vi "FM_Unit_Conversion.vi"(10 "Input Array [A]":dbl[](array[numeric])) -> (2 "Output Array [kg/h]":dbl[](array[numeric]))   [LabVIEW 2017]
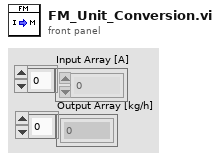
[diagram p1: front panel]
types:
  T1 = cluster{"Input Array [A][0]":dbl, "Input Array [A][1]":dbl, "Input Array [A][2]":dbl, "Input Array [A][3]":dbl}
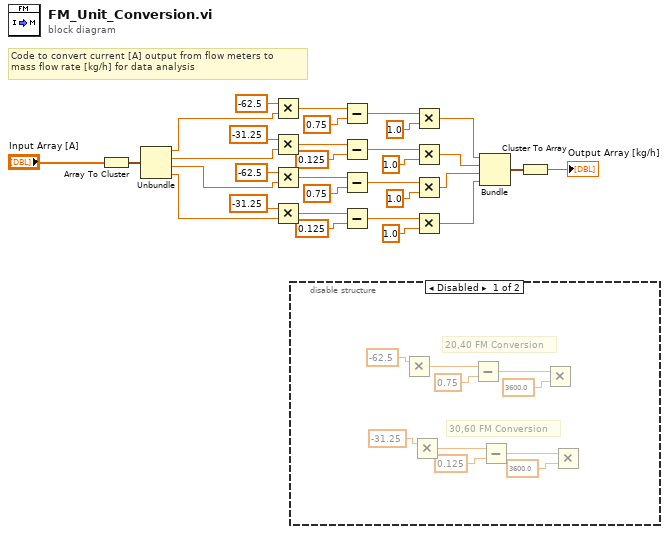
[diagram p0: block diagram]
diagram:
  # "Code to convert current [A] output from flow meters to \nmass flow rate [kg/h] for data analysis"
  n1 = Array To Cluster(array="Input Array [A]") -> (cluster=w32:T1)
  n2 = Unbundle(w32) -> ("Input Array [A][0]"=w9:dbl, "Input Array [A][1]"=w8:dbl, "Input Array [A][2]"=w7:dbl, "Input Array [A][3]"=w6:dbl)
  n3 = Multiply(x=-62.5, y=w9) -> (x*y=w28:dbl)
  n4 = Multiply(x=-31.25, y=w8) -> (x*y=w23:dbl)
  n5 = Multiply(x=-62.5, y=w7) -> (x*y=w18:dbl)
  n6 = Multiply(x=-31.25, y=w6) -> (x*y=w13:dbl)
  n7 = disable-structure shown="Disabled" {
    frame Disabled {
      # "30,60 FM Conversion"
      # "20,40 FM Conversion"
      n8 = Multiply(x=-62.5) -> (x*y=w39:dbl)  [unwired: 1 in]
      n9 = Multiply(x=-31.25) -> (x*y=w41:dbl)  [unwired: 1 in]
      n10 = Subtract(x=w39, y=0.75) -> (x-y=w40:dbl)
      n11 = Subtract(x=w41, y=0.125) -> (x-y=w42:dbl)
      n12 = Multiply(x=w40, y=3600.0) -> ()  [unwired: 1 out]
      n13 = Multiply(x=w42, y=3600.0) -> ()  [unwired: 1 out]
    }
    frame Enabled {
    }
  }
  n14 = Subtract(x=w28, y=0.75) -> (x-y=w26:dbl)
  n15 = Subtract(x=w23, y=0.125) -> (x-y=w21:dbl)
  n16 = Subtract(x=w18, y=0.75) -> (x-y=w16:dbl)
  n17 = Subtract(x=w13, y=0.125) -> (x-y=w11:dbl)
  n18 = Multiply(x=w26, y=1.0) -> (x*y=w2:dbl)
  n19 = Multiply(x=w21, y=1.0) -> (x*y=w3:dbl)
  n20 = Multiply(x=w16, y=1.0) -> (x*y=w4:dbl)
  n21 = Multiply(x=w11, y=1.0) -> (x*y=w5:dbl)
  n22 = Bundle(w2, w3, w4, w5) -> (w31:cluster{dbl, dbl, dbl, dbl})  [unwired: 1 in]
  n23 = Cluster To Array(cluster=w31) -> (array=→"Output Array [kg/h]":dbl[])
